vi "read.vi"(8 "error in":errorcluster, 9 "timeout in ms (-1)":i32=-1, 11 "communicator in":refnum<class "communicator.lvclass">) -> (0 "error out":errorcluster, 1 "timed out?":bool, 2 "message":refnum<class "communicator message.lvclass">)   [LabVIEW 2015, in "communicator.lvclass"]
uses:
  communicator.lvclass
  message/communicator message.lvclass
  communicator.lvclass/communicator.ctl
  communicator queue/identifying queue.lvclass/identifying queue.ctl
  communicator queue/identifying queue.lvclass
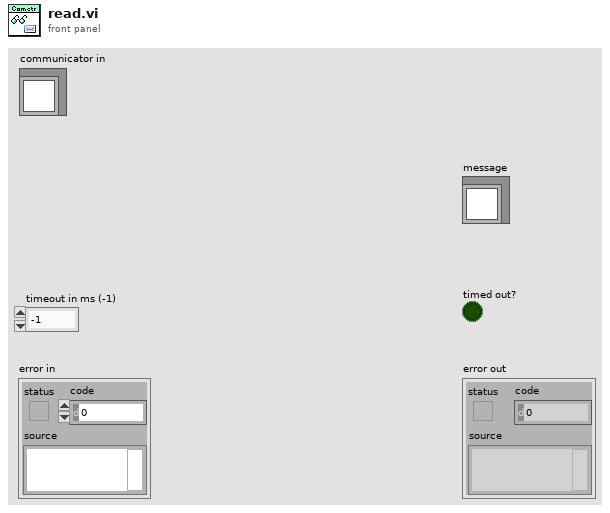
[diagram p1: front panel]
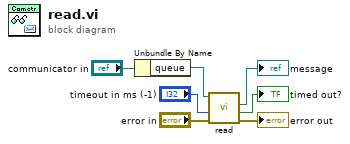
[diagram p0: block diagram]
diagram:
  n1 = Unbundle By Name("communicator in") -> ("queue"=w4:refnum<class "identifying queue.lvclass">)
  n2 = call "read.vi"("error in"="error in", "timeout in ms (-1)"="timeout in ms (-1)", "identifying queue in"=w4) -> ("error out"=→"error out":errorcluster, "timed out?"=→"timed out?":bool, "message"=→"message":refnum<class "communicator message.lvclass">)  [unwired: 6 in]
